vi "pH scale.vi"(2 "V/T":dbl format="%.6f", 3 "pH scale":T1 {"Buffers"."V/T" format="%.5f"; "Buffers"."Buffer" format="%.2f"; "Temperature" format="%.2f"}) -> (0 "number":u32, 1 "pH":dbl format="%.2f")   [LabVIEW 2015]
uses:
  pH scale.ctl
panel:
  # "C"
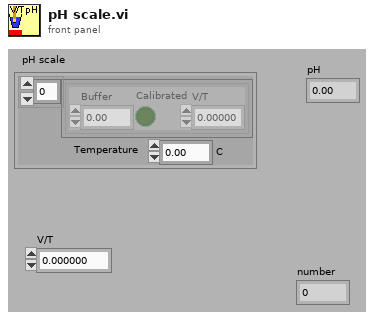
[diagram p1: front panel]
types:
  T1 = typedef "pH scale.ctl" = cluster{"Buffers":cluster{"Buffer":dbl, "Calibrated":bool, "V/T":dbl}[], "Temperature":dbl}
  T2 = cluster{"Buffer":dbl, "Calibrated":bool, "V/T":dbl}[]
  T3 = cluster{"Buffer":dbl, "Calibrated":bool, "V/T":dbl}
  T4 = typedef "correspondence table.ctl" = cluster{"physical units":dbl, "volts":dbl}[]
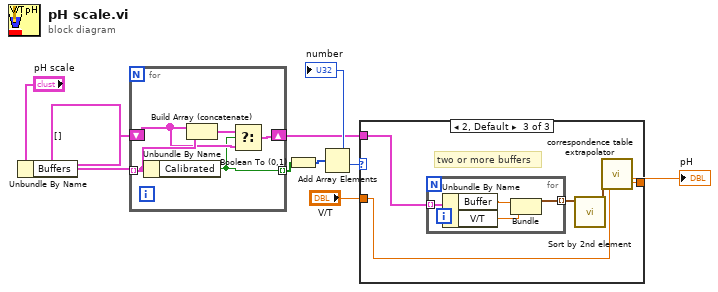
[diagram p0: block diagram]
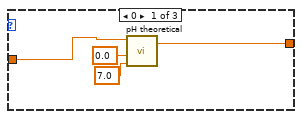
[diagram p2: hidden frame]
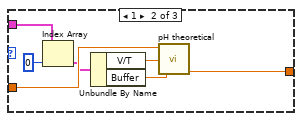
[diagram p3: hidden frame]
diagram:
  n1 = Unbundle By Name("pH scale") -> ("Buffers"=w8:T2)
  n2 = for {
    tunnel: w8 -> [w12] mode=indexing
    tunnel: [w10] -> w7 mode=indexing
    shift-right: [w14] -> w1
    shift-left: T2 [] -> [w11]
    n3 = Unbundle By Name(w12) -> ("Calibrated"=w10:bool)
    n4 = Build Array (concatenate)(w11, w12) -> (w13:T2)
    n5 = Select(t=w13, s=w10, f=w11) -> (s? t:f=w14:T2)
  }
  n6 = Boolean To (0,1)(Boolean=w7) -> (0, 1=w6:i16[])
  n7 = Add Array Elements(numeric array=w6) -> (sum=w5:i16)
  "number" <- w5
  n8 = case shown="2, Default" w5 {
    tunnel: "V/T" -> [w17 w25 w30]
    tunnel: [w18 w19 w29] -> w3
    tunnel: w1 -> [_ w24 w28]
    frame 0 {
      n9 = call "pH theoretical.vi"("pH cal"=7.0, "V/T cal"=0.0, "V/T"=w17) -> ("Theoretical pH"=w18:dbl)  [unwired: 2 in]
    }
    frame 1 {
      n10 = Index Array(array=w24, index=0 ("Index")) -> (element=w22:T3)
      n11 = Unbundle By Name(w22) -> ("V/T"=w21:dbl, "Buffer"=w20:dbl)
      n12 = call "pH theoretical.vi"("pH cal"=w20, "V/T cal"=w21, "V/T"=w25) -> ("Theoretical pH"=w19:dbl)  [unwired: 2 in]
    }
    frame 2, Default {
      # "two or more buffers"
      n13 = for {
        tunnel: w28 -> [w34] mode=indexing
        tunnel: [w31] -> w27 mode=indexing
        n14 = Unbundle By Name(w34) -> ("Buffer"=w33:dbl, "V/T"=w32:dbl)
        n15 = Bundle("Buffer"=w33, "V/T"=w32) -> (w31:cluster{"Buffer":dbl, "V/T":dbl})  [unwired: 1 in]
      }
      n16 = call "Sort by 2nd element.vi"("correspondence table in"=w27) -> ("correspondence table out"=w26:T4)  [unwired: 9 in]
      n17 = call "correspondence table extrapolator.vi"("Volts"=w30, "correspondence table"=w26) -> ("scaled"=w29:dbl)  [unwired: 1 out]
    }
  }
  "pH" <- w3
